vi "Load Reference.vi"(8 "error in (no error)":errorcluster, 10 "Reference":refnum<vi>, 11 "Calendar in":refnum<class "Calendar.lvclass">) -> (0 "error out":errorcluster, 3 "Calendar out":refnum<class "Calendar.lvclass">)   [LabVIEW 2015, in "Calendar.lvclass"]
doc: "The <b>Load Reference VI</b> is a dynamic dispatch VI that must be overwritten in every QControl Class and must <b>Call Parent Method</b>. This recursively loads the reference of the control to the data space for the Control Class up the inheritance hierarchy (class hierarchy). These references must be loaded in this way to use all of the built-in properties.\n\nThe reference input is the reference type needed for the control but is coerced to Generic. It should be cast back to the correct type before bundling into the class private data. The pre-casted \"Generic\" reference is wired as input to the <b>Call Parent Method</b>.\n<b> </b> <b> </b>\n©2016 Q Software Innovations, LLC (QSI)\nwritten by Quentin Alldredge\nproduced in LabVIEW 2015\n\nsupport@qsoftwareinnovations.com\nwww.qsoftwareinnovations.com\n\nAll rights reserved.\n\nRedistribution and use in source and binary forms, with or without modification, are permitted provided that the following conditions are met:\n\n * Redistributions of source code must retain the above copyright notice, this list of conditions and the following disclaimer.\n * Redistributions in binary form must reproduce the above copyright notice, this list of conditions and the following disclaimer in the documentation and/or other materials provided with the distribution.\n * Neither the name of Q Software Innovations, LLC. nor the names of its contributors may be used to endorse or promote products derived from this software without specific prior written permission.\n\nTHIS SOFTWARE IS PROVIDED BY THE COPYRIGHT HOLDERS AND CONTRIBUTORS \"AS IS\" AND ANY EXPRESS OR IMPLIED WARRANTIES, INCLUDING, BUT NOT LIMITED TO, THE IMPLIED WARRANTIES OF MERCHANTABILITY AND FITNESS FOR A PARTICULAR PURPOSE ARE DISCLAIMED. IN NO EVENT SHALL THE COPYRIGHT OWNER OR CONTRIBUTORS BE LIABLE FOR ANY DIRECT, INDIRECT, INCIDENTAL, SPECIAL, EXEMPLARY, OR CONSEQUENTIAL DAMAGES (INCLUDING, BUT NOT LIMITED TO, PROCUREMENT OF SUBSTITUTE GOODS OR SERVICES; LOSS OF USE, DATA, OR PROFITS; OR BUSINESS INTERRUPTION) HOWEVER CAUSED AND ON ANY THEORY OF LIABILITY, WHETHER IN CONTRACT, STRICT LIABILITY, OR TORT (INCLUDING NEGLIGENCE OR OTHERWISE) ARISING IN ANY WAY OUT OF THE USE OF THIS SOFTWARE, EVEN IF ADVISED OF THE POSSIBILITY OF SUCH DAMAGE."
uses:
  Calendar.lvclass
  Calendar.lvclass/Calendar.ctl
  Cluster/Cluster.lvclass
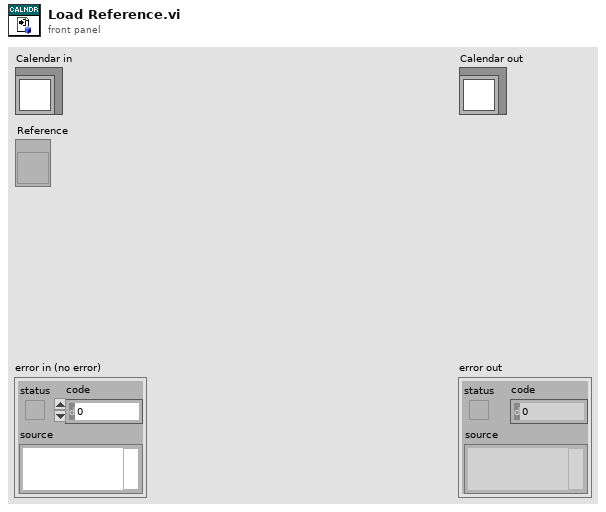
[diagram p1: front panel]
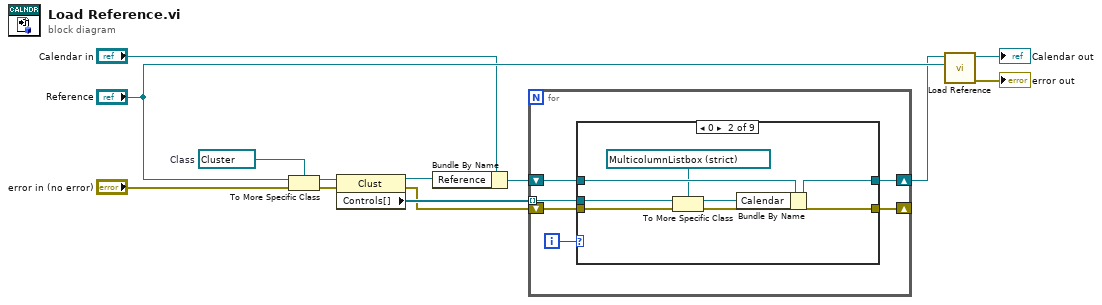
[diagram p0: block diagram]
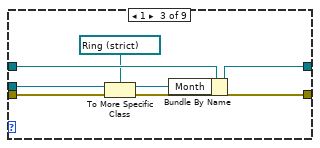
[diagram p3: hidden frame]
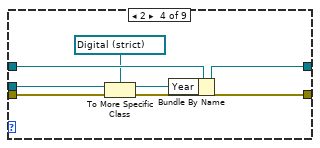
[diagram p4: hidden frame]
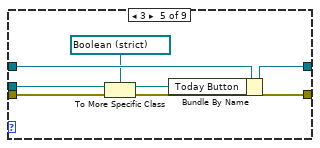
[diagram p5: hidden frame]
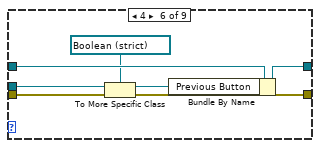
[diagram p6: hidden frame]
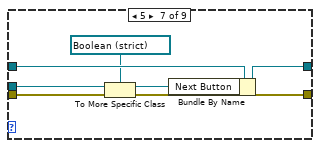
[diagram p7: hidden frame]
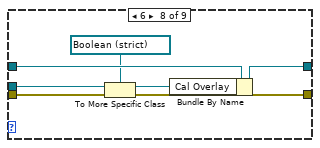
[diagram p8: hidden frame]
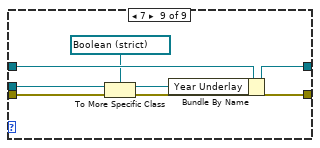
[diagram p9: hidden frame]
diagram:
  w11 = refnum<vi> refnum  # Class
  n1 = To More Specific Class(target class=w11, reference="Reference", error in="error in (no error)") -> (specific class reference=w6:refnum<vi>, error out=w13:errorcluster)
  n2 = property class="Clust"(reference=w6, error in=w13) -> (reference out=w5:refnum<vi>, error out=w1:errorcluster, "Controls[]"=w2:refnum<vi>[])
  n3 = Bundle By Name(cluster="Calendar in", "Reference"=w5) -> (w4:refnum<class "Calendar.lvclass">)
  n4 = for {
    shift-right: [w15] -> w3
    shift-left: w4 -> [w19]
    tunnel: w2 -> [w17] mode=indexing
    shift-right: [w14] -> _
    shift-left: w1 -> [w16]
    i -> [w18]
    n5 = case shown="0" w18 {
      tunnel: w19 -> [w21 w26 w33 w40 w47 w54 w61 w68 w75]
      tunnel: w17 -> [_ w28 w35 w42 w49 w56 w63 w70 w77]
      tunnel: w16 -> [w20 w27 w34 w41 w48 w55 w62 w69 w76]
      tunnel: [w21 w23 w31 w38 w45 w52 w59 w66 w73] -> w15
      tunnel: [w20 w22 w29 w36 w44 w51 w58 w65 w72] -> w14
      frame Default {
      }
      frame 0 {
        n6 = To More Specific Class(target class=refnum<vi> refnum ("Cal"), reference=w28, error in=w27) -> (specific class reference=w25:refnum<vi>, error out=w22:errorcluster)
        n7 = Bundle By Name(cluster=w26, "Calendar"=w25) -> (w23:refnum<class "Calendar.lvclass">)
      }
      frame 1 {
        n8 = To More Specific Class(target class=refnum<vi> refnum ("Month"), reference=w35, error in=w34) -> (specific class reference=w32:refnum<vi>, error out=w29:errorcluster)
        n9 = Bundle By Name(cluster=w33, "Month"=w32) -> (w31:refnum<class "Calendar.lvclass">)
      }
      frame 2 {
        n10 = To More Specific Class(target class=refnum<vi> refnum ("Year"), reference=w42, error in=w41) -> (specific class reference=w39:refnum<vi>, error out=w36:errorcluster)
        n11 = Bundle By Name(cluster=w40, "Year"=w39) -> (w38:refnum<class "Calendar.lvclass">)
      }
      frame 3 {
        n12 = To More Specific Class(target class=refnum<vi> refnum ("Cal Overlay"), reference=w49, error in=w48) -> (specific class reference=w46:refnum<vi>, error out=w44:errorcluster)
        n13 = Bundle By Name(cluster=w47, "Today Button"=w46) -> (w45:refnum<class "Calendar.lvclass">)
      }
      frame 4 {
        n14 = To More Specific Class(target class=refnum<vi> refnum ("Cal Overlay"), reference=w56, error in=w55) -> (specific class reference=w53:refnum<vi>, error out=w51:errorcluster)
        n15 = Bundle By Name(cluster=w54, "Previous Button"=w53) -> (w52:refnum<class "Calendar.lvclass">)
      }
      frame 5 {
        n16 = To More Specific Class(target class=refnum<vi> refnum ("Cal Overlay"), reference=w63, error in=w62) -> (specific class reference=w60:refnum<vi>, error out=w58:errorcluster)
        n17 = Bundle By Name(cluster=w61, "Next Button"=w60) -> (w59:refnum<class "Calendar.lvclass">)
      }
      frame 6 {
        n18 = To More Specific Class(target class=refnum<vi> refnum ("Cal Overlay"), reference=w70, error in=w69) -> (specific class reference=w67:refnum<vi>, error out=w65:errorcluster)
        n19 = Bundle By Name(cluster=w68, "Cal Overlay"=w67) -> (w66:refnum<class "Calendar.lvclass">)
      }
      frame 7 {
        n20 = To More Specific Class(target class=refnum<vi> refnum ("Cal Overlay"), reference=w77, error in=w76) -> (specific class reference=w74:refnum<vi>, error out=w72:errorcluster)
        n21 = Bundle By Name(cluster=w75, "Year Underlay"=w74) -> (w73:refnum<class "Calendar.lvclass">)
      }
    }
  }
  n22 = call-parent "Load Reference.vi"("Reference"="Reference", "Cluster in"=w3) -> ("error out"=→"error out":errorcluster, "Cluster out"=→"Calendar out":refnum<class "Calendar.lvclass">)  [unwired: 8 in]
